vi "Convert number to bytes.vi"(11 "Numeric":dbl) -> (3 "Array":u8[](array[numeric]))   [LabVIEW 2017]
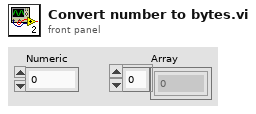
[diagram p1: front panel]
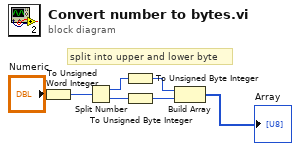
[diagram p0: block diagram]
diagram:
  # "split into upper and lower byte"
  n1 = To Unsigned Word Integer(number="Numeric") -> (unsigned 16bit integer=w6:u16)
  n2 = Split Number(x=w6) -> (hi(x)=w5:u8, lo(x)=w1:u8)
  n3 = To Unsigned Byte Integer(number=w5) -> (unsigned 8bit integer=w2:u8)
  n4 = To Unsigned Byte Integer(number=w1) -> (unsigned 8bit integer=w3:u8)
  n5 = Build Array(w2, w3) -> (→"Array":u8[])
